vi "Field Draw Ball.vi"(4 "Draw Targets?":T2, 6 "balls":T1[](array[typedef]), 8 "picture in":picture, 9 "Offset":T3, 10 "Scale mm/pixel":dbl, 11 "ball":T1) -> (0 "picture out":picture)   [LabVIEW 2018]
uses:
  <vilib>/Utility/miscctls.llb/LVBoundsTypeDef.ctl
  Core/AI Ball.ctl
  DrawTargets.ctl
  <vilib>/Analysis/NI_AALPro.lvlib
  <vilib>/Analysis/coordinate.llb/2D Cartesian Coordinate Rotation (Scalar).vi
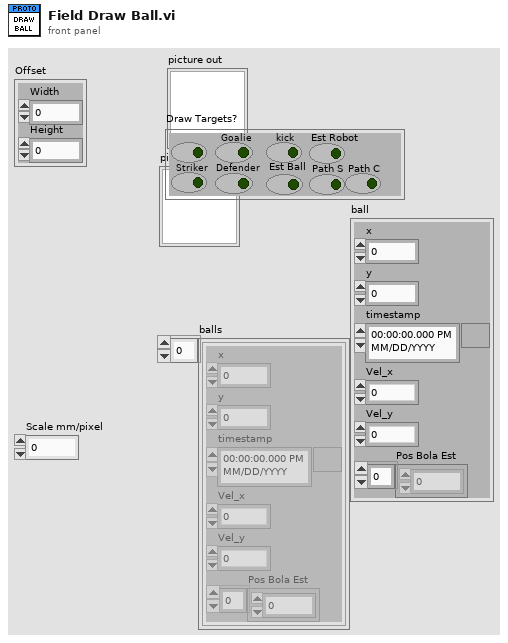
[diagram p1: front panel]
types:
  T1 = typedef "AI Ball.ctl" = cluster{"x":dbl, "y":dbl, "timestamp":timestamp, "Vel_x":dbl, "Vel_y":dbl, "Pos Bola Est":dbl[]}
  T2 = typedef "DrawTargets.ctl" = cluster{"Attacker":bool, "Striker":bool, "Goalie":bool, "Defender":bool, "kick":bool, "Est Ball":bool, "Est Robot":bool, "Path S":bool, "Path C":bool}
  T3 = typedef "LVBoundsTypeDef.ctl" = cluster{"Width":u32, "Height":u32}
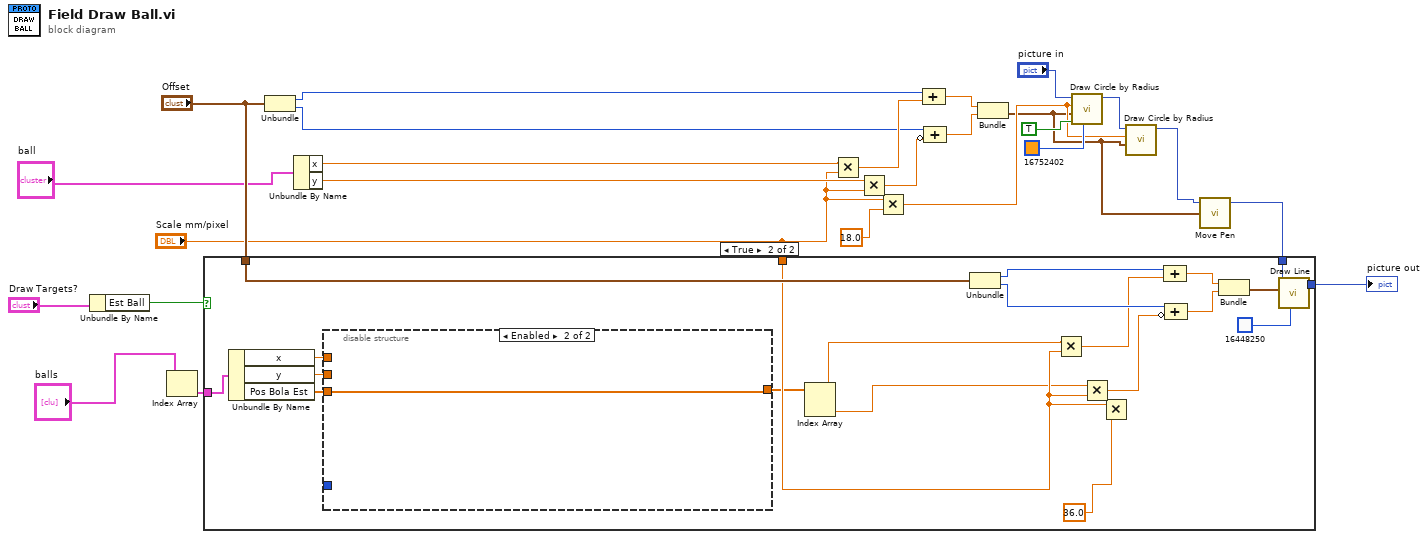
[diagram p0: block diagram]
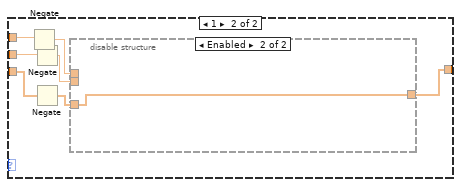
[diagram p4: hidden frame]
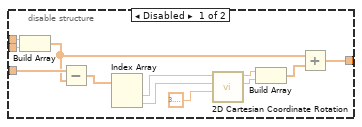
[diagram p5: hidden frame]
diagram:
  n1 = Unbundle By Name("Draw Targets?") -> ("Est Ball"=w2:bool)
  n2 = Index Array(array="balls") -> (element=w4:T1)  [unwired: 1 in]
  n3 = Unbundle("Offset") -> ("Width"=w20:u32, "Height"=w17:u32)
  n4 = Unbundle By Name("ball") -> ("x"=w21:dbl, "y"=w22:dbl)
  n5 = Multiply(x=w21, y="Scale mm/pixel") -> (x*y=w19:dbl)
  n6 = Multiply(x=w22, y="Scale mm/pixel") -> (x*y=w16:dbl)
  n7 = Multiply(x="Scale mm/pixel", y=sgl 18.0 ("radius")) -> (x*y=w12:dbl)
  n8 = Compound Arithmetic op=ADD(w20, w19) -> (w18:dbl)
  n9 = Compound Arithmetic op=ADD(w17, invert w16) -> (w15:dbl)
  n10 = Bundle(w18, w15) -> (w8:cluster{dbl, dbl})  [unwired: 1 in]
  n11 = call <vilib>:"Draw Circle by Radius.vi"("color(black)"=u32 16752402, "fill?(F)"=TRUE, "pixel center"=w8, "radius"=w12, "picture"="picture in") -> ("new picture"=w13:picture)  [unwired: 6 in]
  n12 = call <vilib>:"Draw Circle by Radius.vi"("pixel center"=w8, "radius"=w12, "picture"=w13) -> ("new picture"=w9:picture)  [unwired: 8 in]
  n13 = call <vilib>:"Move Pen.vi"("new position"=w8, "picture"=w9) -> ("new picture"=w10:picture)  [unwired: 3 in]
  n14 = case shown="True" w2 {
    tunnel: [w26 w46] -> w11
    tunnel: w10 -> [w26 w45]
    tunnel: "Offset" -> [_ w40]
    tunnel: "Scale mm/pixel" -> [_ w37]
    tunnel: w4 -> [_ w34]
    frame False {
    }
    frame True {
      n15 = Unbundle By Name(w34) -> ("x"=w28:dbl, "y"=w27:dbl, "Pos Bola Est"=w30:dbl[])
      n16 = disable-structure shown="Enabled" {
        disable-tunnel: _ -> [w51 _]
        disable-tunnel: w30 -> [w50 w73]
        disable-tunnel: [w49 w73] -> w29
        disable-tunnel: w28 -> [w48 _]
        disable-tunnel: w27 -> [w47 _]
        frame Disabled {
          n17 = case shown="0, Default" w51 {
            tunnel: [w52 w53] -> w49
            tunnel: w50 -> [w52 w56]
            tunnel: w48 -> [_ w55]
            tunnel: w47 -> [_ w54]
            frame 0, Default {
            }
            frame 1 {
              n18 = Negate(x=w55) -> (-x=w59:dbl)
              n19 = Negate(x=w54) -> (-x=w58:dbl)
              n20 = Negate(x=w56) -> (-x=w57:dbl[])
              n21 = disable-structure shown="Enabled" {
                disable-tunnel: w59 -> [w66 _]
                disable-tunnel: w58 -> [w65 _]
                disable-tunnel: w57 -> [w64 w72]
                disable-tunnel: [w60 w72] -> w53
                frame Disabled {
                  n22 = Build Array(w66, w65) -> (w61:dbl[])
                  n23 = Subtract(x=w64, y=w61) -> (x-y=w63:dbl[])
                  n24 = Index Array(array=w63) -> (element #1=w71:dbl, element #2=w70:dbl)  [unwired: 2 in]
                  n25 = call-poly <vilib>:"2D Cartesian Coordinate Rotation.vi"("theta"=3.141592653589793, "y"=w70, "x"=w71) -> ("y out"=w68:dbl, "x out"=w69:dbl)  [unwired: 6 in, 1 out]
                  n26 = Build Array(w69, w68) -> (w62:dbl[])
                  n27 = Add(x=w61, y=w62) -> (x+y=w60:dbl[])
                }
                frame Enabled {
                }
              }
            }
          }
        }
        frame Enabled {
        }
      }
      n28 = Index Array(array=w29) -> (element #1=w33:dbl, element #2=w32:dbl)  [unwired: 2 in]
      n29 = Unbundle(w40) -> ("Width"=w44:u32, "Height"=w42:u32)
      n30 = Multiply(x=w33, y=w37) -> (x*y=w36:dbl)
      n31 = Multiply(x=w32, y=w37) -> (x*y=w35:dbl)
      n32 = Multiply(x=w37, y=sgl 36.0 ("radius")) -> ()  [unwired: 1 out]
      n33 = Compound Arithmetic op=ADD(w44, w36) -> (w43:dbl)
      n34 = Compound Arithmetic op=ADD(w42, invert w35) -> (w41:dbl)
      n35 = Bundle(w43, w41) -> (w39:cluster{dbl, dbl})  [unwired: 1 in]
      n36 = call <vilib>:"Draw Line.vi"("picture"=w45, "end point"=w39, "color(black)"=u32 16448250) -> ("new picture"=w46:picture)  [unwired: 6 in]
    }
  }
  "picture out" <- w11
